vi "Autonomous Independent.vi"() -> ()   [LabVIEW 2014]
doc: "This VI is called when autonomous begins, and will automatically be terminated when autonomous ends. You can carry out timed or sensor driven robot movement independently without needing to return to the caller."
uses:
  <vilib>/Rock Robotics/WPI/Joystick/WPI_JoystickGetSetRefNum.vi
  <vilib>/Rock Robotics/Network Tables/SD Write Numeric Array.vi
  <vilib>/Rock Robotics/WPI/RobotDrive/WPI_RobotDriveGetSetRefNum.vi
  <vilib>/Rock Robotics/WPI/RobotDrive/WPI_RobotDriveMecanumDrive_Cartesian.vi
panel:
  out "Current Movement, for debugging":T1 {"Z Joystick Value" scale=-1.0..1.0; "Y Joystick Value" scale=1.0..-1.0; "X Joystick Value" scale=-1.0..1.0}
  in  "Array of robot movements":T2(array[cluster]) {"Z Joystick Value" scale=-1.0..1.0; "Y Joystick Value" scale=1.0..-1.0; "X Joystick Value" scale=-1.0..1.0}
  # "Be sure to right-click and choose Data Operations>>Make Current Value default if you want to save the array values with the VI"
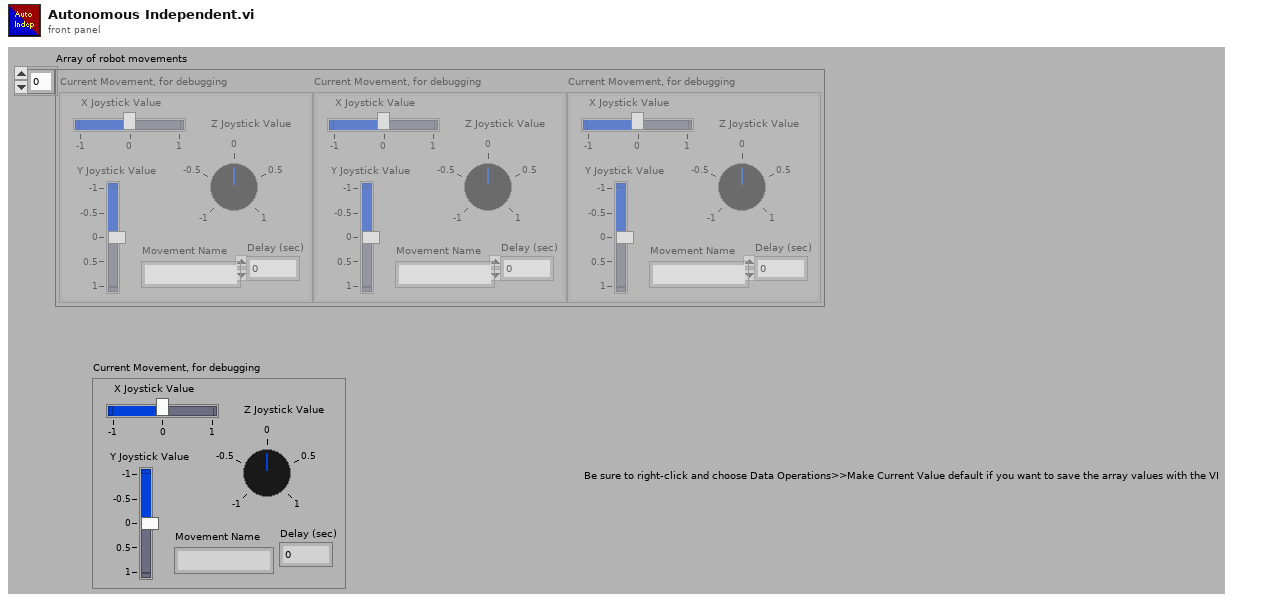
[diagram p1: front panel]
types:
  T1 = cluster{"X Joystick Value":dbl, "Y Joystick Value":dbl, "Z Joystick Value":dbl, "Delay (sec)":dbl, "Movement Name":string}
  T2 = cluster{"X Joystick Value":dbl, "Y Joystick Value":dbl, "Z Joystick Value":dbl, "Delay (sec)":dbl, "Movement Name":string}[]
  T3 = typedef "WPI_JoystickDevRef.ctl" = cluster{"Device":T4}
  T4 = typedef "WPI_JoystickDeviceEnum.ctl" = enum16{"USB 0", "USB 1", "USB 2", "USB 3", "USB 4", "USB 5"}
  T5 = typedef "WPI_RobotDriveDevRef.ctl" = cluster{"DevStatus":errorcluster, "Motors[]":T6[], "Square Inputs":bool, "Max Output":dbl}
  T6 = typedef "WPI_MotorControlDeviceRef.ctl" = cluster{"DeviceStatus":errorcluster, "Type":T7, "PWM":cluster{"Controller":T8, "PWM Channel":T9, "DeadBand":T10}, "CAN":cluster{"Device Number":u8, "Control Mode":T11, "Semaphore":T12, "Max Vout":dbl, "TalonSRX Control Mode":T13}, "Invert":bool, "TransformRef":T14, "InvTransformRef":T14}
  T7 = typedef "WPI_MotorControlType.ctl" = enum16{"PWM", "CAN", "CANTalonSRX"}
  T8 = typedef "FPGA_TypedefDigitalModule.ctl" = enum16{"Controller 1"}
  T9 = typedef "FPGA_DIOPWMChannel.ctl" = enum8{"PWM 0", "PWM 1", "PWM 2", "PWM 3", "PWM 4", "PWM 5", "PWM 6", "PWM 7", "PWM 8", "PWM 9", "PWM MXP 0", "PWM MXP 1", "PWM MXP 2", "PWM MXP 3", "PWM MXP 4", "PWM MXP 5", "PWM MXP 6", "PWM MXP 7", "PWM MXP 8", "PWM MXP 9", "Invalid"}
  T10 = typedef "WPI_PWMDeadband.ctl" = cluster{"Name":string, "maxPositivePwm":i32, "minPositivePwm":i32, "centerPwm":i32, "maxNegativePwm":i32, "minNegativePwm":i32, "angularRange":u16}
  T11 = typedef "WPI_CANJaguar_ControlMode.ctl" = enum8{"Percent VBus", "Current", "Speed", "Position", "Voltage"}
  T12 = typedef "Semaphore RefNum" = refnum<k1>
  T13 = typedef "WPI_CANTalonSRX_APIControlMode.ctl" = enum8{"Percent VBus", "Speed", "Position", "Slave", "Unchanged / Invalid"}
  T14 = typedef "WPI_PWMTransform_ConPane.ctl" = refnum<vi>
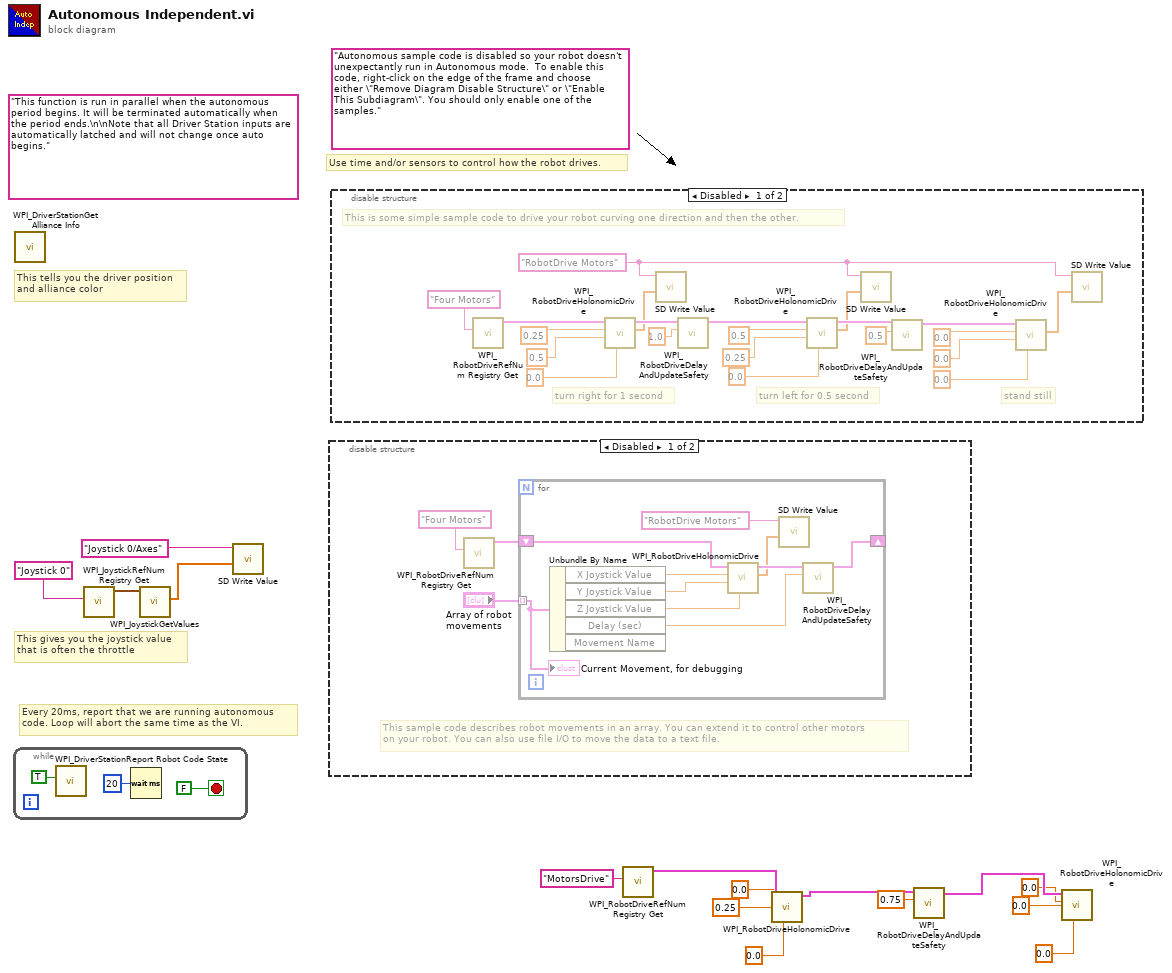
[diagram p0: block diagram]
diagram:
  (unwired) "Autonomous sample code is disabled so your robot doesn't unexpectantly run in Autonomous mode.  To enable this code, right-click on the edge of the frame and choose either \"Remove Diagram Disable Structure\" or \"Enable This Subdiagram\". You should only enable one of the samples."
  (unwired) "This function is run in parallel when the autonomous period begins. It will be terminated automatically when the period ends.\n\nNote that all Driver Station inputs are automatically latched and will not change once auto begins."
  # "Every 20ms, report that we are running autonomous\ncode. Loop will abort the same time as the VI."
  # "This gives you the joystick value\nthat is often the throttle"
  # "Use time and/or sensors to control how the robot drives."
  # "This tells you the driver position\nand alliance color"
  n1 = while {
    stop <- FALSE stop-if-true
    n2 = call <vilib>:"WPI_DriverStationReport Robot Code State.vi"("Autonomous"=TRUE) -> ()  [unwired: 10 in, 1 out]
    n3 = Wait (ms)(milliseconds to wait=u32 20) -> ()  [unwired: 1 out]
  }
  n4 = call <vilib>:"WPI_DriverStationGet Alliance Info.vi"() -> ()  [unwired: 12 out]
  n5 = call <vilib>:"WPI_JoystickRefNum Registry Get.vi"("refnum name"="Joystick 0") -> ("JoystickDevRef"=w14:T3)  [unwired: 1 in, 9 out]
  n6 = call <vilib>:"WPI_JoystickGetValues.vi"("JoystickDevRef"=w14) -> ("Axes"=w12:dbl[])  [unwired: 6 in, 4 out]
  n7 = call-poly <vilib>:"SD Write Value.vi"("Numeric Array"=w12, "Name"="Joystick 0/Axes") -> ()  [unwired: 8 in, 2 out]
  n8 = disable-structure shown="Disabled" {
    frame Disabled {
      # "This sample code describes robot movements in an array. You can extend it to control other motors\non your robot. You can also use file I/O to move the data to a text file."
      n9 = call <vilib>:"WPI_RobotDriveRefNum Registry Get.vi"("refnum name"="Four Motors") -> ("RobotDriveDevRef"=w20:T5)  [unwired: 1 in, 9 out]
      n10 = for {
        shift-right: [w28] -> _
        shift-left: w20 -> [w29]
        tunnel: "Array of robot movements" -> [w25] mode=indexing
        n11 = Unbundle By Name(w25) -> ("X Joystick Value"=w27:dbl, "Y Joystick Value"=w26:dbl, "Z Joystick Value"=w24:dbl, "Delay (sec)"=w22:dbl)  [unwired: 1 out]
        n12 = call-poly <vilib>:"WPI_RobotDriveHolonomicDrive.vi"("Rotation"=w24, "Y"=w26, "X"=w27, "RobotDriveDevRef"=w29) -> ("Motor Values"=w23:dbl[], "RobotDriveDevRef"=w30:T5)  [unwired: 5 in, 1 out]
        n13 = call-poly <vilib>:"SD Write Value.vi"("Numeric Array"=w23, "Name"="RobotDrive Motors") -> ()  [unwired: 8 in, 2 out]
        n14 = call <vilib>:"WPI_RobotDriveDelayAndUpdateSafety.vi"("Delay (s)"=w22, "RobotDriveDevRef"=w30) -> ("RobotDriveDevRef 2"=w28:T5)  [unwired: 8 in, 1 out]
        "Current Movement, for debugging" <- w25
      }
    }
    frame Enabled {
    }
  }
  n15 = disable-structure shown="Disabled" {
    frame Disabled {
      w38 = "RobotDrive Motors" ("Name")
      # "This is some simple sample code to drive your robot curving one direction and then the other."
      # "stand still"
      # "turn left for 0.5 second"
      # "turn right for 1 second"
      n16 = call <vilib>:"WPI_RobotDriveRefNum Registry Get.vi"("refnum name"="Four Motors") -> ("RobotDriveDevRef"=w39:T5)  [unwired: 1 in, 9 out]
      n17 = call-poly <vilib>:"WPI_RobotDriveHolonomicDrive.vi"("Rotation"=0.0, "Y"=0.5 ("X axis value"), "X"=0.25 ("X axis value"), "RobotDriveDevRef"=w39) -> ("Motor Values"=w34:dbl[], "RobotDriveDevRef"=w46:T5)  [unwired: 5 in, 1 out]
      n18 = call-poly <vilib>:"SD Write Value.vi"("Numeric Array"=w34, "Name"=w38) -> ()  [unwired: 8 in, 2 out]
      n19 = call <vilib>:"WPI_RobotDriveDelayAndUpdateSafety.vi"("Delay (s)"=1.0, "RobotDriveDevRef"=w46) -> ("RobotDriveDevRef 2"=w45:T5)  [unwired: 8 in, 1 out]
      n20 = call-poly <vilib>:"WPI_RobotDriveHolonomicDrive.vi"("Rotation"=0.0, "Y"=0.25 ("X axis value"), "X"=0.5 ("X axis value"), "RobotDriveDevRef"=w45) -> ("Motor Values"=w33:dbl[], "RobotDriveDevRef"=w44:T5)  [unwired: 5 in, 1 out]
      n21 = call-poly <vilib>:"SD Write Value.vi"("Numeric Array"=w33, "Name"=w38) -> ()  [unwired: 8 in, 2 out]
      n22 = call <vilib>:"WPI_RobotDriveDelayAndUpdateSafety.vi"("Delay (s)"=0.5, "RobotDriveDevRef"=w44) -> ("RobotDriveDevRef 2"=w43:T5)  [unwired: 8 in, 1 out]
      n23 = call-poly <vilib>:"WPI_RobotDriveHolonomicDrive.vi"("Rotation"=0.0 ("X axis value"), "Y"=0.0 ("X axis value"), "X"=0.0 ("X axis value"), "RobotDriveDevRef"=w43) -> ("Motor Values"=w32:dbl[])  [unwired: 5 in, 2 out]
      n24 = call-poly <vilib>:"SD Write Value.vi"("Numeric Array"=w32, "Name"=w38) -> ()  [unwired: 8 in, 2 out]
    }
    frame Enabled {
    }
  }
  n25 = call <vilib>:"WPI_RobotDriveRefNum Registry Get.vi"("refnum name"="MotorsDrive") -> ("RobotDriveDevRef"=w10:T5)  [unwired: 9 in, 1 out]
  n26 = call-poly <vilib>:"WPI_RobotDriveHolonomicDrive.vi"("Rotation"=0.0, "Y"=0.25, "X"=0.0, "RobotDriveDevRef"=w10) -> ("RobotDriveDevRef"=w7:T5)  [unwired: 5 in, 2 out]
  n27 = call <vilib>:"WPI_RobotDriveDelayAndUpdateSafety.vi"("Delay (s)"=0.75, "RobotDriveDevRef"=w7) -> ("RobotDriveDevRef 2"=w2:T5)  [unwired: 8 in, 1 out]
  n28 = call-poly <vilib>:"WPI_RobotDriveHolonomicDrive.vi"("Rotation"=0.0, "Y"=0.0, "X"=0.0, "RobotDriveDevRef"=w2) -> ()  [unwired: 5 in, 3 out]
